vi "DQMH Set Modules.vi"(7 "Module Disk Path":path, 8 "error in (no error)":errorcluster, 10 "modules to load dynamically":path[](array[path]), 11 "Application reference":refnum<vi>) -> (0 "error out":errorcluster)   [LabVIEW 2020, in "hse-dqmh-dynamicrequesters.lvlib"]
doc: "Calls the \"Set Modules\" request VI of the module in <b>Path to module directory</b>. Hands over paths to all dynamically loaded modules in <b>modules to load dynamically</b>.\n\n____\nHAMPEL SOFTWARE ENGINEERING v3.8.0 (2023-12-18 14:41)"
uses:
  hse-dqmh-dynamicrequesters.lvlib
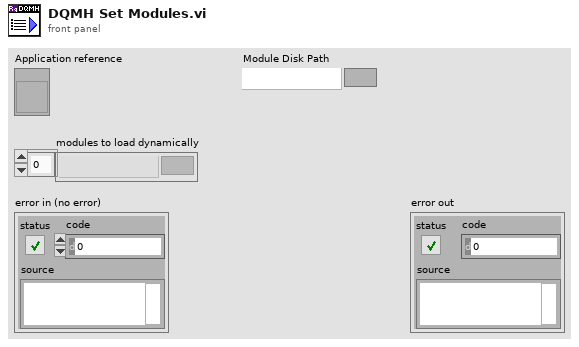
[diagram p1: front panel]
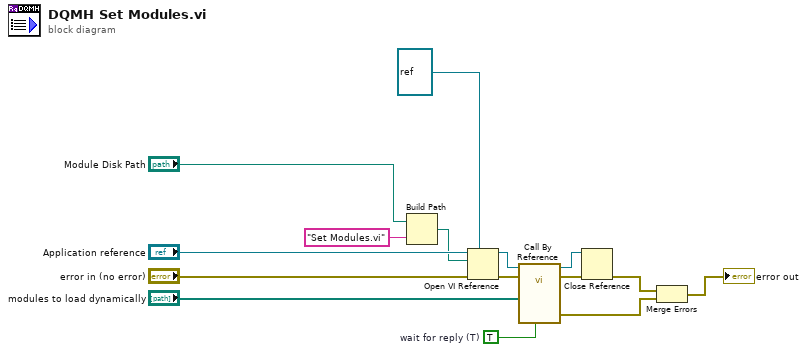
[diagram p0: block diagram]
diagram:
  w1 = TRUE  # wait for reply (T)
  n1 = Build Path(base path="Module Disk Path", name or relative path="Set Modules.vi") -> (appended path=w10:path)
  n2 = Open VI Reference(type specifier VI Refnum (for type only)=refnum<vi> refnum, application reference (local)="Application reference", vi path=w10, error in (no error)="error in (no error)") -> (vi reference=w13:refnum<vi>, error out=w7:errorcluster)  [unwired: 2 in]
  n3 = call-by-ref "?"(reference=w13, error in=w7, "wait for reply (T)"=w1, "Module Paths"="modules to load dynamically") -> (reference out=w3:refnum<vi>, error out=w8:errorcluster, 0:"error out"=w9:errorcluster)  [unwired: 8 in, 1 out]
  n4 = Close Reference(reference=w3, error in (no error)=w8) -> (error out=w4:errorcluster)
  n5 = Merge Errors(w4, w9) -> (→"error out":errorcluster)
